vi "DL950_wave2.vi"() -> ()   [LabVIEW 2019]
uses:
  _ctrl/cDAQ-9269 Config.ctl
  _ctrl/DL950_config.ctl
  _ctrl/init-r-stop.ctl
  _ctrl/create-rw-close.ctl
  _ctrl/rw.ctl
  _ctrl/start.ctl
panel:
  in  "DL950_Stop":bool
  in  "DL950_Read":bool
  in  "탭 컨트롤":enum32{"DL950", "AO"}(tab)
  in  "config":T1={"Timeout"=10000, "Time Div"=19, "Acq Mode"=0, "Record Len"=5, "Record Num"=0, "Start Point"=0, "End Poin"=60000, "Visa"="TCPIP0::192.168.0.100::inst0::INSTR", "Config Voltage"=[{"Enable"=TRUE, "Ch"=0, "V Div"=12, "Coupling"=1, "Probe"=3, "Act.Items"=FALSE, "items"=[]}, {"Enable"=TRUE, "Ch"=0, "V Div"=12, "Coupling"=1, "Probe"=3, "Act.Items"=FALSE, "items"=[]}, {"Enable"=FALSE, "Ch"=0, "V Div"=20, "Coupling"=1, "Probe"=3, "Act.Items"=FALSE, "items"=[]}, {"Enable"=FALSE, "Ch"=0, "V Div"=20, "Coupling"=1, "Probe"=3, "Act.Items"=FALSE, "items"=[]}, {"Enable"=FALSE, "Ch"=0, "V Div"=20, "Coupling"=1, "Probe"=3, "Act.Items"=FALSE, "items"=[]}, {"Enable"=FALSE, "Ch"=0, "V Div"=20, "Coupling"=1, "Probe"=3, "Act.Items"=FALSE, "items"=[]}], "Trigger on"=FALSE, "Trigger Level"=0.0, "Reset"=FALSE, "Config Temp"=[], "Trigger Mode"=1, "Trigger Position"=50.0, "Trigger Slope"=0, "Trigger Source "=1, "Start Point (-5.00)"=-5.0, "End Point (5.00)"=5.0} {"End Point (5.00)" format="%.2g"; "Start Point (-5.00)" format="%.2f"; "Trigger Source" items=["", "CH1", "CH2", "CH3", "CH4", "CH5", "CH6", "CH7", "CH8", "CH9", "CH10", "CH11", "CH12", "CH13", "CH14", "CH15", "CH16", "RMATH1", "RMATH2", "RMATH3", "RMATH4", "RMATH5", "RMATH6", "RMATH7", "RMATH8", "RMATH9", "RMATH10", "RMATH11", "RMATH12", "RMATH13", "RMATH14", "RMATH15", "RMATH16"]; "Trigger Slope" items=["Rising", "Falling", "Both"]; "Trigger Position" format="%.1f"; "Trigger Mode" items=["Normal", "Auto", "Auto Level", "Single", "Single(N)", "On Start", "No Set"]; "Config Temp"."Type" items=["K", "E", "J", "T", "L", "U", "N", "R", "S", "B", "W", "Au7fe"]; "Config Temp"."Channel" items=["", "CH1", "CH2", "CH3", "CH4", "CH5", "CH6", "CH7", "CH8", "CH9", "CH10", "CH11", "CH12", "CH13", "CH14", "CH15", "CH16"]; "Trigger Level" format="%.3p"; "Config Voltage"."items" items=["Peak to Peak", "Amplitude", "Max", "Min", "High", "Low", "Average", "Middle", "Rms", "Standard Deviation", "+Overshoot", "-Overshoot", "Rise", "Fall", "Frequency", "Period", "+Width", "-Width", "Duty Cycle", "Pulse Count", "Burst1 Width", "Burst2 Width", "Average Frequency", "Average Period", "Int1TY", "Int2TY"]; "Config Voltage"."Probe" items=["1:1", "2:1", "5:1", "10:1", "20:1", "50:1", "100:1", "200:1", "500:1", "1000:1", "2000:1", "5000:1", "10k:1", "20k:1", "50k:1", "0.1A:1V", "0.2A:1V", "0.5A:1V", "1A:1V", "2A:1V", "5A:1V", "10A:1V", "20A:1V", "50A:1V", "100A:1V", "200A:1V", "250A:1V", "400A:1V", "500A:1V", "1kA:1V", "2kA:1V", "5kA:1V", "10kA:1V", "20kA:1V", "50kA:1V", "NoSet"]; "Config Voltage"."Ch" items=["None", "CH1", "CH2", "CH3", "CH4", "CH5", "CH6", "CH7", "CH8", "CH9", "CH10", "CH11", "CH12", "CH13", "CH14", "CH15", "CH16", "MATH1", "MATH2", "MATH3", "MATH4", "MATH5", "MATH6", "MATH7", "MATH8", "EVENT"]; "Config Voltage"."Coupling" items=["AC", "DC", "Ground", "AC-RMS", "DC-RMS"]; "Config Voltage"."V Div" items=["0.1m", "0.2m", "0.5m", "1m", "2m", "5m", "10m", "20m", "50m", "100m", "200m", "500m", "1", "2", "4", "5", "8", "10", "20", "40", "50", "80", "100", "200", "400", "500", "800", "1k", "2k", "4k", "5k", "8k", "10k", "20k", "25k", "50k", "100k", "250k", "500k", "1000k"]; "Record Len" items=["10k", "25k", "50k", "100k", "250k", "500k", "1M", "2.5M", "5M", "10M", "25M", "50M", "100M", "250M", "500M", "1G", "2G", "4G", "5G", "10G", "20G", "50G"]; "Acq Mode" items=["Normal", "Average", "Envelope"]; "Time Div" items=["100ns", "200ns", "500ns", "1us", "2us", "5us", "10us", "20us", "50us", "100us", "200us", "500us", "1ms", "2ms", "5ms", "10ms", "20ms", "50ms", "100ms", "200ms", "500ms", "1s", "2s", "3s", "4s", "5s", "6s", "10s", "20s", "30s", "1min", "2min", "3min", "4min", "5min", "6min", "10min", "12min", "30min", "1hour", "2hour", "3hour", "4hour", "5hour", "6hour", "8hour", "10hour", "12hour", "1day", "2day", "3day", "4day", "5day"]}
  in  "DL950_Apply":bool
  out "ch1 graph":waveform(dbl)(graph)={"t0"=timestamp(0 s since 1904-01-01), "dt"=5e-07, "Y"=array[10001 elements]}
  out "ch2 graph":waveform(dbl)(graph)={"t0"=timestamp(0 s since 1904-01-01), "dt"=5e-07, "Y"=array[10001 elements]}
  in  "Config_AO":T2={"Ch"="cDAQ1Mod1/ao0", "Max V"=5.0, "Min V"=-5.0, " Rate"=1000.0, "N pts"=100, "sample mode"=0} {"sample mode" items=["유한 샘플"=10178, "연속 샘플"=10123, "하드웨어 타이밍에 의한 단일 포인트"=12522]}
  in  "AO signal":T3={"offset"=1.0, "signal type"=enum."Square Wave", "frequency"=10.0, "amplitude"=1.0, " duty"=50.0} {"amplitude" format="%0.2p"; "frequency" format="%.0p"; "offset" format="%0.2p"}
  in  "DL950_Check":bool
  in  "DL950_DisConnect":bool
  in  "DL950_Connect":bool
  in  "DL950_Start":bool
  in  "Exit":bool
  in  "Stop":bool
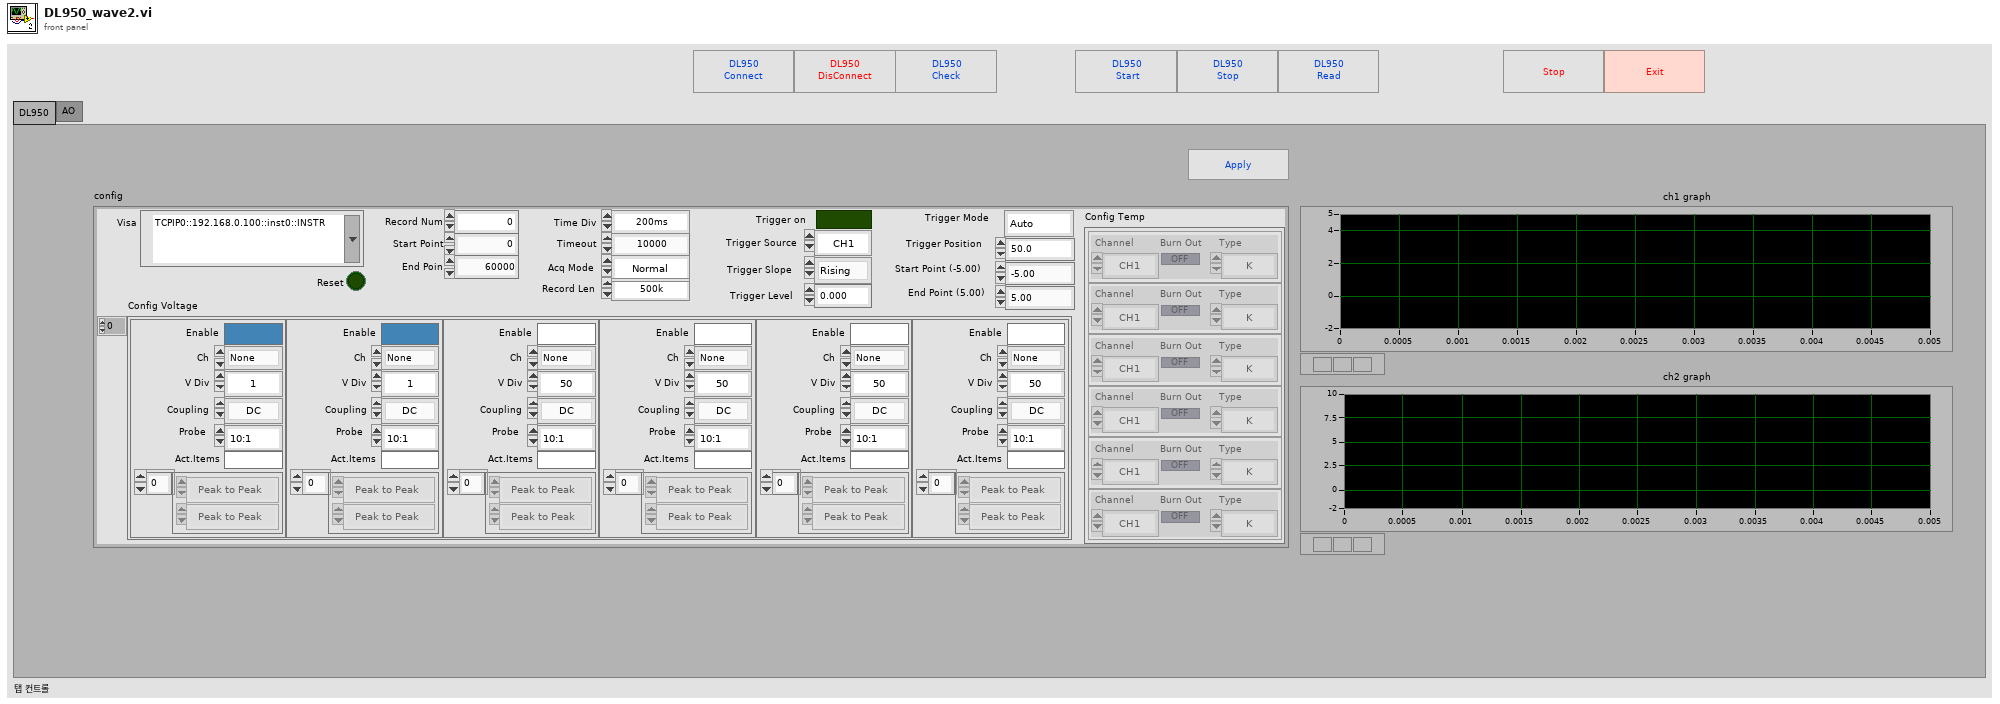
[diagram p1: front panel]
types:
  T1 = typedef "DL950_config.ctl" = cluster{"Timeout":u32, "Time Div":i32, "Acq Mode":i32, "Record Len":i32, "Record Num":i32, "Start Point":i64, "End Poin":i64, "Visa":refnum<visa-resource-name>, "Config Voltage":cluster{"Enable":bool, "Ch":u16, "V Div":i32, "Coupling":i32, "Probe":i32, "Act.Items":bool, "items":i32[]}[], "Trigger on":bool, "Trigger Level":dbl, "Reset":bool, "Config Temp":cluster{"Channel":u16, "Burn Out":bool, " Type ":i32}[], "Trigger Mode":i32, "Trigger Position":dbl, "Trigger Slope":i32, "Trigger Source ":i32, "Start Point (-5.00)":dbl, "End Point (5.00)":dbl}
  T2 = typedef "cDAQ-9269 Config.ctl" = cluster{"Ch":tag, "Max V":dbl, "Min V":dbl, " Rate":dbl, "N pts":i32, "sample mode":i32}
  T3 = cluster{"offset":dbl, "signal type":enum16{"Sine Wave", "Triangle Wave", "Square Wave", "Sawtooth Wave"}, "frequency":dbl, "amplitude":dbl, " duty":dbl}
  T4 = typedef "create-rw-close.ctl" = enum16{"create", "write", "read", "close"}
  T5 = typedef "init-r-stop.ctl" = enum16{"ini", "read", "stop"}
  T6 = typedef "rw.ctl" = enum16{"read", "write"}
  T7 = typedef "start.ctl" = enum16{"init", "open", "set", "start", "stop", "read", "read_items", "query", "close", "T_single", "reset", "exit"}
  T8 = typedef "DL950_wfms.ctl" = cluster{"wfms":waveform(dbl)[], "Waveform_2":cluster{"t0":dbl, "dt":dbl, "Y":dbl[][]}, "items":dbl[][]}
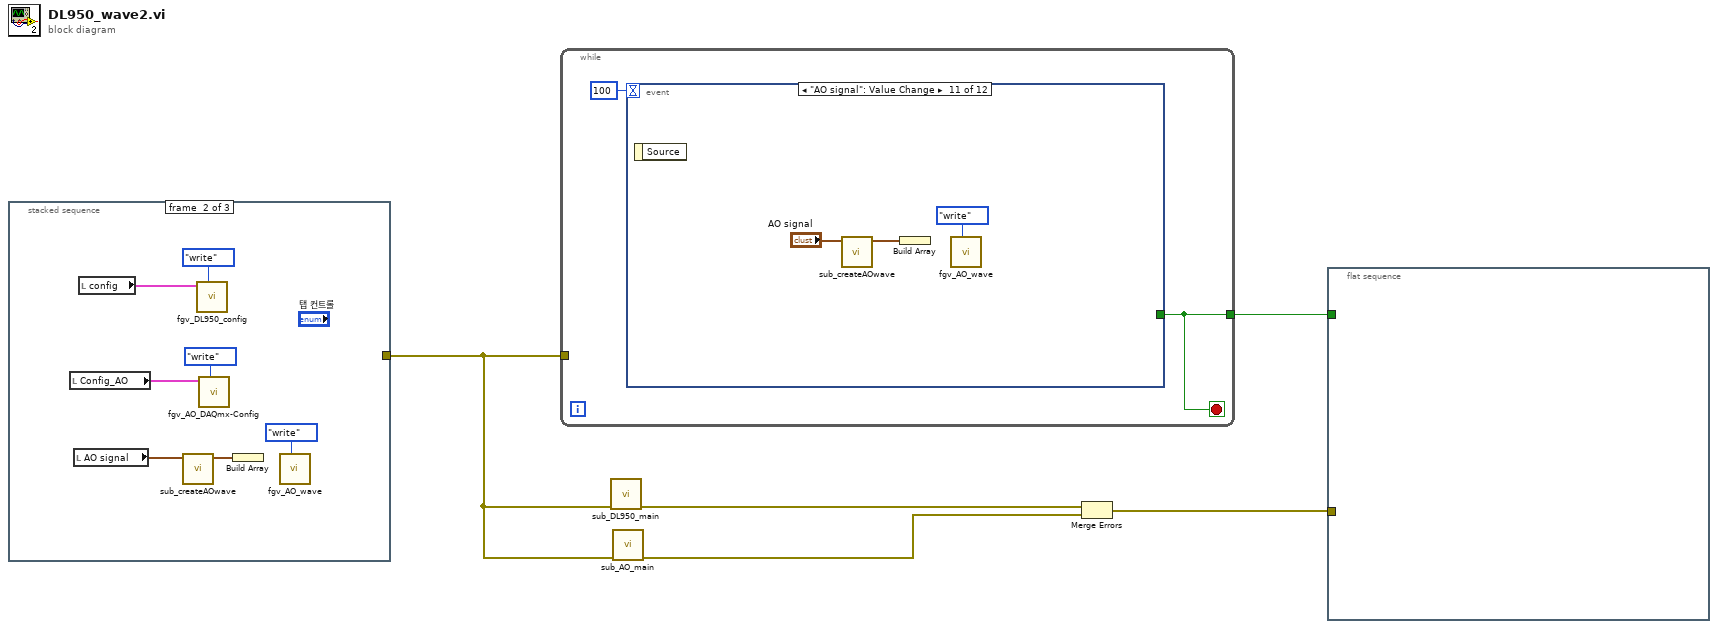
[diagram p0: block diagram]
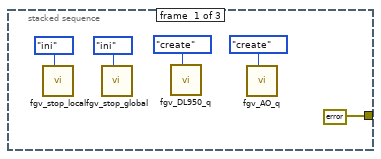
[diagram p2: hidden frame]
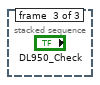
[diagram p3: hidden frame]
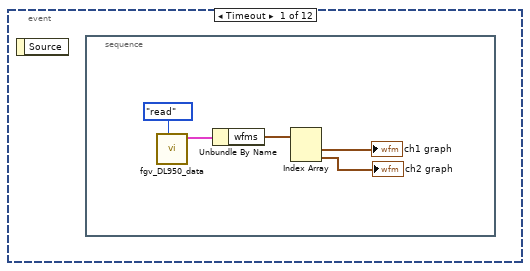
[diagram p4: hidden frame]
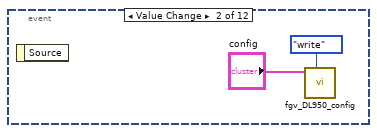
[diagram p5: hidden frame]
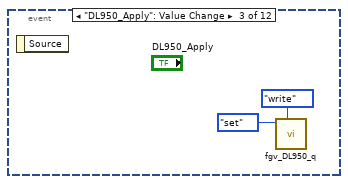
[diagram p6: hidden frame]
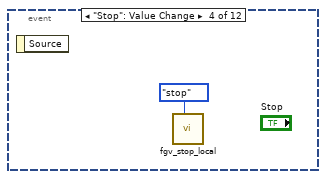
[diagram p7: hidden frame]
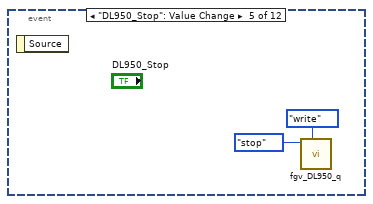
[diagram p8: hidden frame]
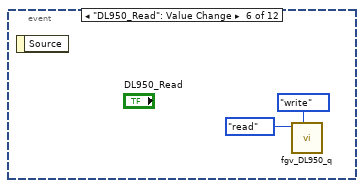
[diagram p9: hidden frame]
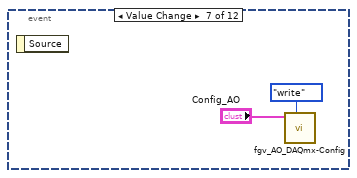
[diagram p10: hidden frame]
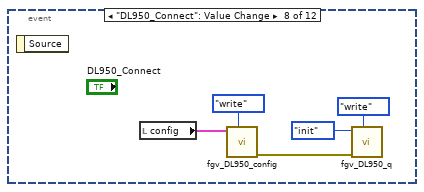
[diagram p11: hidden frame]
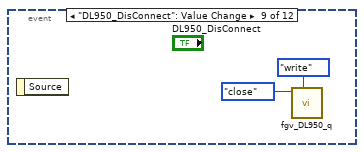
[diagram p12: hidden frame]
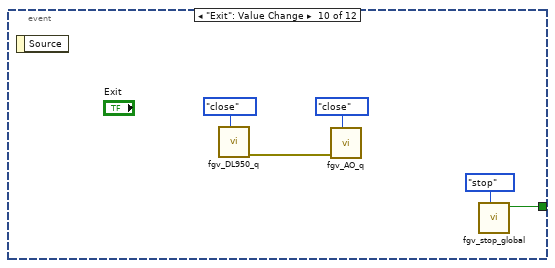
[diagram p13: hidden frame]
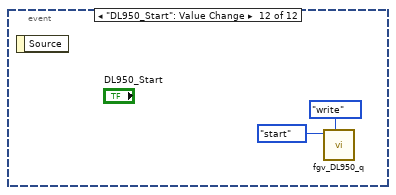
[diagram p14: hidden frame]
diagram:
  n1 = stacked-sequence {
    tunnel: [errorcluster {"status"=FALSE, "code"=0, "source"=""} ("에러 상수") _ _] -> w2
    frame #0 {
      n2 = call "fgv_stop_local.vi"("cmd"=init-r-stop."ini") -> ()  [unwired: 10 in, 1 out]
      n3 = call "fgv_stop_global.vi"("cmd"=init-r-stop."ini") -> ()  [unwired: 10 in, 1 out]
      n4 = call "fgv_DL950_q.vi"("cmd"=create-rw-close."create") -> ()  [unwired: 9 in, 2 out]
      n5 = call "fgv_AO_q.vi"("cmd"=create-rw-close."create") -> ()  [unwired: 9 in, 2 out]
    }
    frame #1 {
      n6 = local read "Config_AO"() -> (w14:T2)
      n7 = local read "AO signal"() -> (w13:T3)
      n8 = local read "config"() -> (w16:T1)
      n9 = call "sub_createAOwave.vi"("AO signal"=w13) -> ("AO wave"=w11:waveform(dbl))  [unwired: 10 in]
      n10 = call "fgv_DL950_config.vi"("cmd"=rw."write", "config"=w16) -> ()  [unwired: 8 in, 2 out]
      n11 = call "fgv_AO_DAQmx-Config.vi"("cmd"=rw."write", "9269 AO Config"=w14) -> ()  [unwired: 8 in, 2 out]
      n12 = Build Array(w11) -> ()  [unwired: 1 out]
      n13 = call "fgv_AO_wave.vi"("cmd"=rw."write") -> ()  [unwired: 9 in, 2 out]
    }
    frame #2 {
    }
  }
  n14 = while {
    tunnel: w2 -> [_]
    tunnel: [w19] -> w5
    stop <- w19 stop-if-true
    n15 = event shown="[10] \"AO signal\": Value Change" {
      selector: _ -> [_ _ _ _ _ _ _ _ _ _ _ _]
      dyn-events: _ -> [_ _ _ _ _ _ _ _ _ _ _ _]
      timeout: 100 -> [_ _ _ _ _ _ _ _ _ _ _ _]
      tunnel: [_ _ _ _ _ _ _ _ _ w46 _ _] -> w19
      event Timeout {
        n16 = event-data() -> ()  [unwired: 1 in, 1 out]
        n17 = stacked-sequence {
          frame #0 {
            n18 = call "fgv_DL950_data.vi"("cmd"=rw."read") -> ("DL950 wfm 2"=w21:T8)  [unwired: 9 in, 1 out]
            n19 = Unbundle By Name(w21) -> ("wfms"=w20:waveform(dbl)[])
            n20 = Index Array(array=w20) -> (element #1=→"ch1 graph":waveform(dbl), element #2=→"ch2 graph":waveform(dbl))  [unwired: 2 in]
          }
        }
      }
      event Value Change {
        n21 = event-data() -> ()  [unwired: 1 in, 1 out]
        n22 = call "fgv_DL950_config.vi"("cmd"=rw."write", "config"="config") -> ()  [unwired: 8 in, 2 out]
      }
      event "DL950_Apply": Value Change {
        n23 = event-data() -> ()  [unwired: 1 in, 1 out]
        n24 = call "fgv_DL950_q.vi"("cmd"=create-rw-close."write", "data"=start."set") -> ()  [unwired: 8 in, 2 out]
      }
      event "Stop": Value Change {
        n25 = event-data() -> ()  [unwired: 1 in, 1 out]
        n26 = call "fgv_stop_local.vi"("cmd"=init-r-stop."stop") -> ()  [unwired: 10 in, 1 out]
      }
      event "DL950_Stop": Value Change {
        n27 = event-data() -> ()  [unwired: 1 in, 1 out]
        n28 = call "fgv_DL950_q.vi"("cmd"=create-rw-close."write", "data"=start."stop") -> ()  [unwired: 8 in, 2 out]
      }
      event "DL950_Read": Value Change {
        n29 = event-data() -> ()  [unwired: 1 in, 1 out]
        n30 = call "fgv_DL950_q.vi"("cmd"=create-rw-close."write", "data"=start."read") -> ()  [unwired: 8 in, 2 out]
      }
      event Value Change {
        n31 = event-data() -> ()  [unwired: 1 in, 1 out]
        n32 = call "fgv_AO_DAQmx-Config.vi"("cmd"=rw."write", "9269 AO Config"="Config_AO") -> ()  [unwired: 8 in, 2 out]
      }
      event "DL950_Connect": Value Change {
        n33 = event-data() -> ()  [unwired: 1 in, 1 out]
        n34 = local read "config"() -> (w38:T1)
        n35 = call "fgv_DL950_config.vi"("cmd"=rw."write", "config"=w38) -> ("error out"=w36:errorcluster)  [unwired: 8 in, 1 out]
        n36 = call "fgv_DL950_q.vi"("cmd"=create-rw-close."write", "error in"=w36, "data"=start."init") -> ()  [unwired: 7 in, 2 out]
      }
      event "DL950_DisConnect": Value Change {
        n37 = event-data() -> ()  [unwired: 1 in, 1 out]
        n38 = call "fgv_DL950_q.vi"("cmd"=create-rw-close."write", "data"=start."close") -> ()  [unwired: 8 in, 2 out]
      }
      event "Exit": Value Change {
        n39 = event-data() -> ()  [unwired: 1 in, 1 out]
        n40 = call "fgv_DL950_q.vi"("cmd"=create-rw-close."close") -> ("error out"=w43:errorcluster)  [unwired: 9 in, 1 out]
        n41 = call "fgv_AO_q.vi"("cmd"=create-rw-close."close", "error in"=w43) -> ()  [unwired: 8 in, 2 out]
        n42 = call "fgv_stop_global.vi"("cmd"=init-r-stop."stop") -> ("stop"=w46:bool)  [unwired: 10 in]
      }
      event "AO signal": Value Change {
        n43 = event-data() -> ()  [unwired: 1 in, 1 out]
        n44 = call "sub_createAOwave.vi"("AO signal"="AO signal") -> ("AO wave"=w50:waveform(dbl))  [unwired: 10 in]
        n45 = Build Array(w50) -> ()  [unwired: 1 out]
        n46 = call "fgv_AO_wave.vi"("cmd"=rw."write") -> ()  [unwired: 9 in, 2 out]
      }
      event "DL950_Start": Value Change {
        n47 = event-data() -> ()  [unwired: 1 in, 1 out]
        n48 = call "fgv_DL950_q.vi"("cmd"=create-rw-close."write", "data"=start."start") -> ()  [unwired: 8 in, 2 out]
      }
    }
  }
  n49 = call "sub_DL950_main.vi"("error in"=w2) -> ("error out"=w4:errorcluster)  [unwired: 9 in, 1 out]
  n50 = call "sub_AO_main.vi"("error in"=w2) -> ("error out"=w1:errorcluster)  [unwired: 10 in]
  n51 = Merge Errors(w4, w1) -> (w3:errorcluster)
  n52 = flat-sequence {
    tunnel: w5 -> [_]
    tunnel: w3 -> [_]
    frame #0 {
    }
  }
